vi "Ping Sift Proxy.vi"(0 "Sift Client in":refnum<class "Sift Client.lvclass">, 7 "Timeout":i32, 11 "error in (no error)":errorcluster) -> (4 "Sift Client out":refnum<class "Sift Client.lvclass">, 6 "Success":bool, 15 "error out":errorcluster)   [LabVIEW 2024, in "Sift Client.lvlib" / "Sift Client.lvclass"]
doc: "Pings Sift Proxy."
uses:
  Sift Client.lvclass
  Sift Client.lvclass/Sift Client.ctl
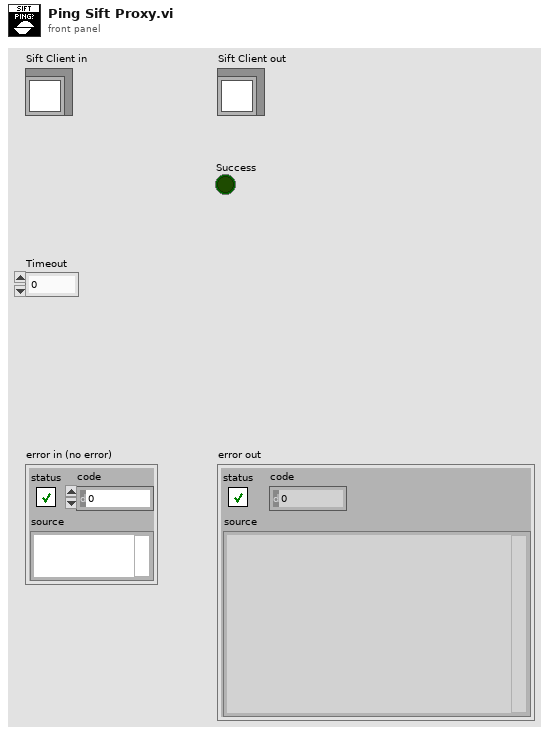
[diagram p1: front panel]
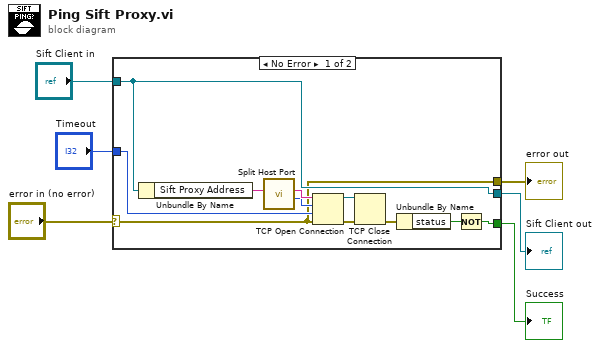
[diagram p0: block diagram]
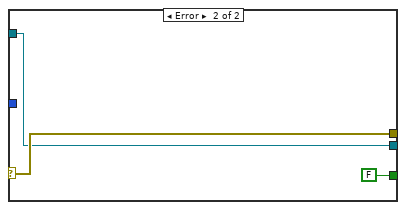
[diagram p2: hidden frame]
diagram:
  n1 = case shown="No Error" "error in (no error)" {
    selector: "error in (no error)" -> [w7 w20]
    tunnel: [w7 w20] -> w5
    tunnel: [w15 w19] -> w3
    tunnel: "Sift Client in" -> [w15 w19]
    tunnel: [w14 FALSE] -> w2
    tunnel: "Timeout" -> [w16 _]
    frame No Error {
      n2 = Unbundle By Name(w15) -> ("Sift Proxy Address"=w10:string)
      n3 = call "Split Host Port.vi"("Address"=w10) -> ("Port"=w8:i32, "Hostname"=w9:string)  [unwired: 9 in]
      n4 = TCP Open Connection(address=w9, remote port or service name=w8, timeout ms (60000)=w16, error in (no error)=w7) -> (connection ID=w12:refnum<k5>, error out=w11:errorcluster)  [unwired: 1 in]
      n5 = TCP Close Connection(connection ID=w12, error in (no error)=w11) -> (error out=w13:errorcluster)  [unwired: 1 in, 1 out]
      n6 = Unbundle By Name(w13) -> ("status"=w17:bool)
      n7 = Not(x=w17) -> (.not. x?=w14:bool)
    }
    frame Error {
    }
  }
  "error out" <- w5
  "Sift Client out" <- w3
  "Success" <- w2
